vi "Process Inputs.vi"(10 "Command Inputs":T1, 11 "Sensor Inputs":T9) -> (3 "OutputsCluster":T16)   [LabVIEW 2012]
uses:
  Outputs_All.ctl
  Flywheel/Outputs_Flywheel.ctl
  tankdrive/Output_Wheel_Speeds.ctl
  Conveyor/Conveyor_outputs.ctl
  Conveyor/Conveyor module state.ctl
  Conveyor/Conveyor_outputsV2.ctl
  Conveyor/3-Ball-Conveyor_Module_State.ctl
  Conveyor/T_Roller module state.ctl
  Turret/Outputs_Turret.ctl
  Roller/Outputs_Roller.ctl
  Bridge Tipper/Outputs_Tipper.ctl
  Inputs_All.ctl
  Flywheel/Sensor_Inputs_FlyWheel.ctl
  tankdrive/Input_Sensors_Drive.ctl
  Conveyor/Sensor_Input_Conveyor.ctl
  Conveyor/Sensor_Input_ConveyorV2.ctl
  Turret/Inputs_Sensors_Turret.ctl
  Inputs_Camera.ctl
  Command_Inputs.ctl
  tankdrive/Input_Commands_Drive.ctl
  Conveyor/Input_Command_Conveyor.ctl
  Turret/Inputs_Commands_Turret.ctl
  Bridge Tipper/Inputs_Tipper.ctl
  Dashboard Controls.ctl
  Roller/Input_Commands_Roller.ctl
  Flywheel/Input_Commands_Flywheel.ctl
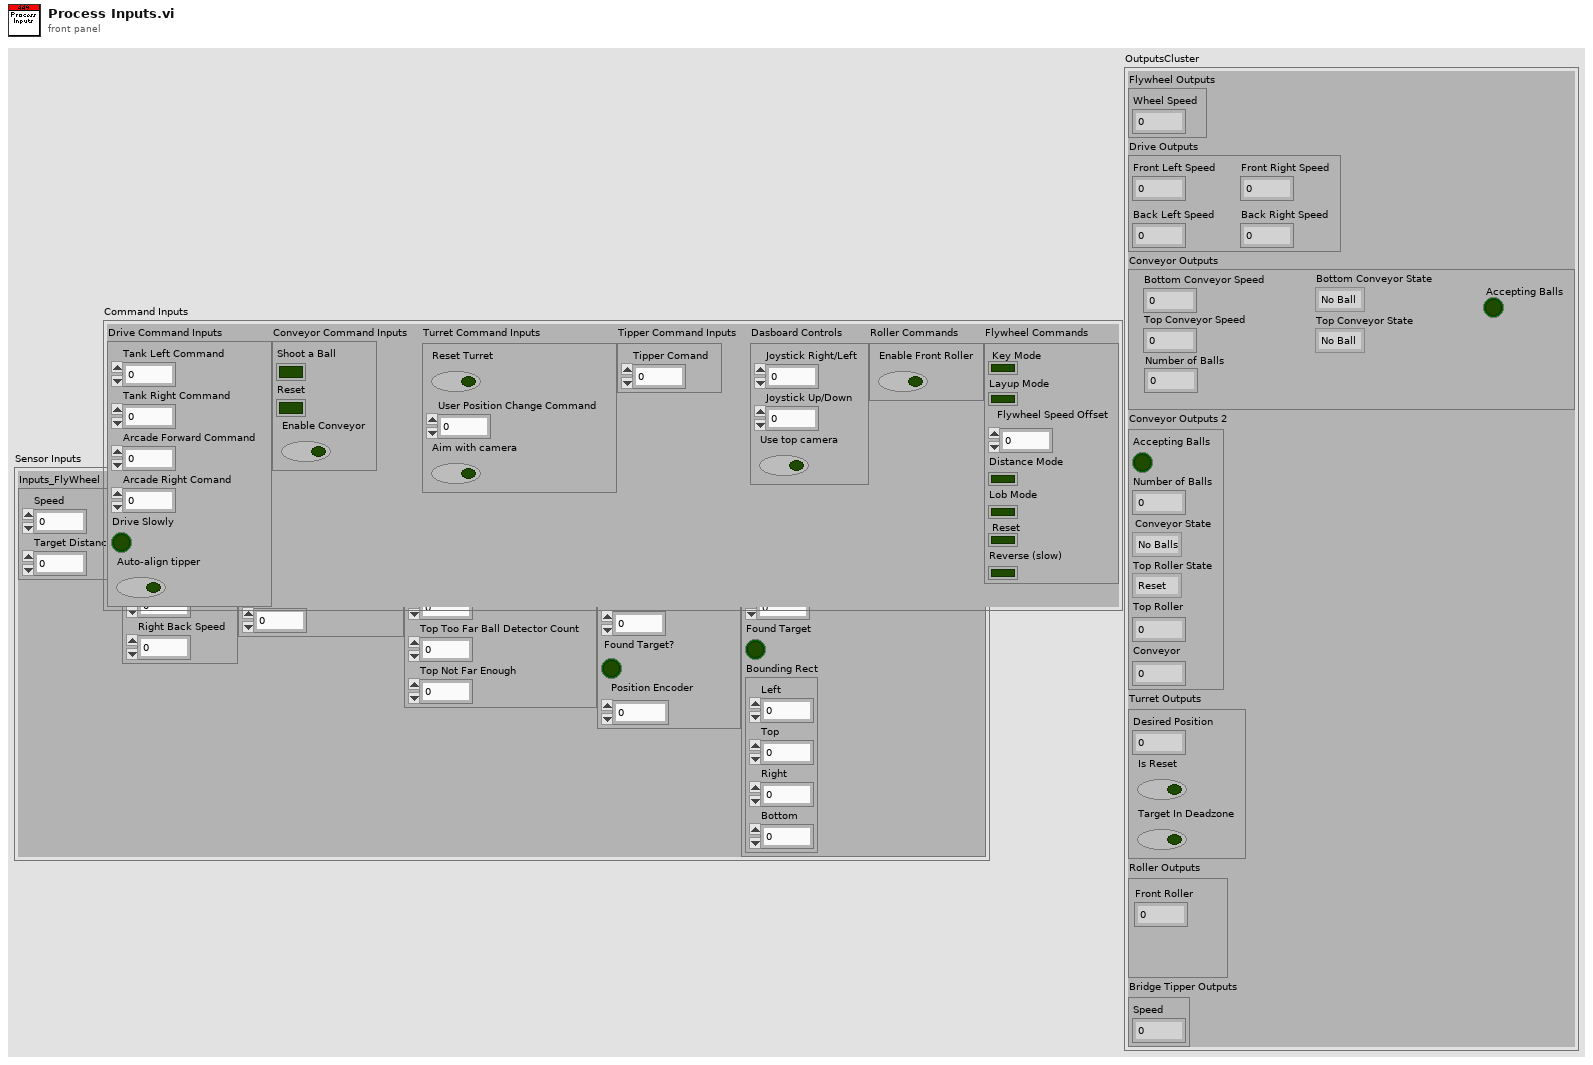
[diagram p1: front panel]
types:
  T1 = typedef "Command_Inputs.ctl" = cluster{"Drive Command Inputs":T2, "Conveyor Command Inputs":T3, "Turret Command Inputs":T4, "Tipper Command Inputs":T5, "Dasboard Controls":T6, "Roller Commands":T7, "Flywheel Commands":T8}
  T2 = typedef "Input_Commands_Drive.ctl" = cluster{"Tank Left Command":dbl, "Tank Right Command":dbl, "Arcade Forward Command":dbl, "Arcade Right Comand":dbl, "Drive Slowly":bool, "Auto-align tipper":bool}
  T3 = typedef "Input_Command_Conveyor.ctl" = cluster{"Shoot a Ball":bool, "Reset":bool, "Enable Conveyor":bool}
  T4 = typedef "Inputs_Commands_Turret.ctl" = cluster{"Reset Turret":bool, "User Position Change Command":dbl, "Aim with camera":bool}
  T5 = typedef "Inputs_Tipper.ctl" = cluster{"Tipper Comand":dbl}
  T6 = typedef "Dashboard Controls.ctl" = cluster{"Joystick Right/Left":dbl, "Joystick Up/Down":dbl, "Use top camera":bool}
  T7 = typedef "Input_Commands_Roller.ctl" = cluster{"Enable Front Roller":bool}
  T8 = typedef "Input_Commands_Flywheel.ctl" = cluster{"Key Mode":bool, "Layup Mode":bool, "Flywheel Speed Offset":dbl, "Distance Mode":bool, "Lob Mode":bool, "Reset":bool, "Reverse (slow)":bool}
  T9 = typedef "Inputs_All.ctl" = cluster{"Inputs_FlyWheel":T10, "Drive Inputs":T11, "Conveyor Inputs":T12, "ConveyorV2 Inputs":T13, "Turret Inputs":T14, "Camera Inputs":T15}
  T10 = typedef "Sensor_Inputs_FlyWheel.ctl" = cluster{"Speed":dbl, "Target Distance":dbl}
  T11 = typedef "Input_Sensors_Drive.ctl" = cluster{"Left Front Speed":dbl, "Right Front Speed":dbl, "Left Back Speed":dbl, "Right Back Speed":dbl}
  T12 = typedef "Sensor_Input_Conveyor.ctl" = cluster{"Top Ball Detector Count":i32, "Bottom Ball Detector Count":i32, "Shooter Ball Detector Count":i32}
  T13 = typedef "Sensor_Input_ConveyorV2.ctl" = cluster{"Grab Ball Detector Count":i32, "Bottom Ball Detector Count":i32, "Top In Place Ball Detector Count":i32, "Top Too Far Ball Detector Count":i32, "Top Not Far Enough":i32}
  T14 = typedef "Inputs_Sensors_Turret.ctl" = cluster{"At Minimum Angle":bool, "At Maximum Angle":bool, "Camera Position Offset":dbl, "Found Target?":bool, "Position Encoder":dbl}
  T15 = typedef "Inputs_Camera.ctl" = cluster{"Offset Angle from Perpendicular (degrees)":dbl, "Target Dist":dbl, "Elevation Angle":dbl, "Found Target":bool, "Bounding Rect":cluster{"Left":dbl, "Top":dbl, "Right":dbl, "Bottom":dbl}}
  T16 = typedef "Outputs_All.ctl" = cluster{"Flywheel Outputs":T17, "Drive Outputs":T18, "Conveyor Outputs":T19, "Conveyor Outputs 2":T21, "Turret Outputs":T24, "Roller Outputs":T25, "Bridge Tipper Outputs":T26}
  T17 = typedef "Outputs_Flywheel.ctl" = cluster{"Wheel Speed":dbl}
  T18 = typedef "Output_Wheel_Speeds.ctl" = cluster{"Front Left Speed":dbl, "Front Right Speed":dbl, "Back Left Speed":dbl, "Back Right Speed":dbl}
  T19 = typedef "Conveyor_outputs.ctl" = cluster{"Bottom Conveyor Speed":dbl, "Top Conveyor Speed":dbl, "Bottom Conveyor State":T20, "Top Conveyor State":T20, "Accepting Balls":bool, "Number of Balls":i32}
  T20 = typedef "Conveyor module state.ctl" = enum16{"No Ball", "Has Ball", "Ball Below Hold", "Ball Above Hold", "Outputting Ball", "Reset"}
  T21 = typedef "Conveyor_outputsV2.ctl" = cluster{"Accepting Balls":bool, "Number of Balls":i32, "Conveyor State":T22, "Top Roller State":T23, "Top Roller":dbl, "Conveyor":dbl}
  T22 = typedef "3-Ball-Conveyor_Module_State.ctl" = enum16{"No Balls", "Collecting Ball", "Holding 1", "Pushing Ball Out", "Holding 2", "Lowering Ball", "Reset", "Disabled"}
  T23 = typedef "T_Roller module state.ctl" = enum16{"Reset", "Disabled", "Waiting for Ball", "Holding", "Ball not far enough", "Ball too far", "Firing"}
  T24 = typedef "Outputs_Turret.ctl" = cluster{"Desired Position":dbl, "Is Reset":bool, "Target In Deadzone":bool}
  T25 = typedef "Outputs_Roller.ctl" = cluster{"Front Roller":dbl}
  T26 = typedef "Outputs_Tipper.ctl" = cluster{"Speed":dbl}
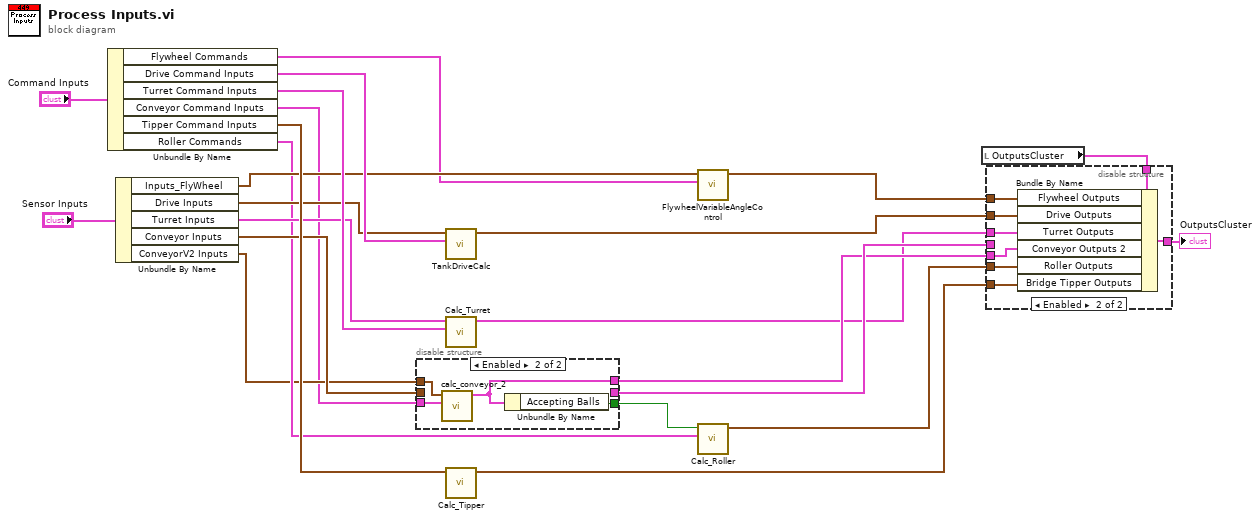
[diagram p0: block diagram]
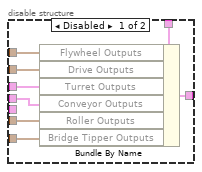
[diagram p2: hidden frame]
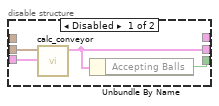
[diagram p3: hidden frame]
diagram:
  n1 = Unbundle By Name("Command Inputs") -> ("Flywheel Commands"=w7:T8, "Drive Command Inputs"=w17:T2, "Turret Command Inputs"=w19:T4, "Conveyor Command Inputs"=w2:T3, "Tipper Command Inputs"=w22:T5, "Roller Commands"=w6:T7)
  n2 = Unbundle By Name("Sensor Inputs") -> ("Inputs_FlyWheel"=w14:T10, "Drive Inputs"=w15:T11, "Turret Inputs"=w18:T14, "Conveyor Inputs"=w20:T12, "ConveyorV2 Inputs"=w5:T13)
  n3 = disable-structure shown="Enabled" {
    disable-tunnel: [w25 _] -> w23
    disable-tunnel: w2 -> [w27 w31]
    disable-tunnel: w20 -> [w26 _]
    disable-tunnel: w5 -> [_ w30]
    disable-tunnel: [_ w29] -> w3
    disable-tunnel: [w24 w28] -> w4
    frame Disabled {
      n4 = call "calc_conveyor.vi"("Conveyor Command Inputs"=w27, "Conveyor Sensor Inputs"=w26) -> ("Conveyor Outputs"=w25:T19)  [unwired: 9 in]
      n5 = Unbundle By Name(w25) -> ("Accepting Balls"=w24:bool)
    }
    frame Enabled {
      n6 = call "calc_conveyor_2.vi"("Conveyor Command Inputs"=w31, "ConveyorV2 Inputs"=w30) -> ("Conveyor Outputs"=w29:T21)  [unwired: 9 in]
      n7 = Unbundle By Name(w29) -> ("Accepting Balls"=w28:bool)
    }
  }
  n8 = call "TankDriveCalc.vi"("Drive Command Inputs"=w17, "Drive Sensor Inputs"=w15) -> ("Drive Outputs"=w10:T18)  [unwired: 9 in]
  n9 = call "Calc_Turret.vi"("Turret Command Inputs"=w19, "Turret Sensor Inputs"=w18) -> ("Turret Outputs"=w1:T24)  [unwired: 9 in]
  n10 = call "Calc_Tipper.vi"("Tipper Command Inputs"=w22) -> ("Bridge Tipper Outputs"=w13:T26)  [unwired: 10 in]
  n11 = call "FlywheelVariableAngleControl.vi"("Flywheel Commands"=w7, "Inputs_FlyWheel"=w14) -> ("Outputs_Flywheel"=w9:T17)  [unwired: 9 in]
  n12 = call "Calc_Roller.vi"("Roller Commands"=w6, "Accepting Balls?"=w4) -> ("Roller Outputs"=w12:T25)  [unwired: 9 in]
  n13 = local read "OutputsCluster"() -> (w8:T16)
  n14 = disable-structure shown="Enabled" {
    disable-tunnel: w1 -> [w39 w43]
    disable-tunnel: w23 -> [w38 _]
    disable-tunnel: w13 -> [w37 w41]
    disable-tunnel: w12 -> [w36 w42]
    disable-tunnel: [w35 w47] -> w11
    disable-tunnel: w10 -> [w34 w44]
    disable-tunnel: w9 -> [w33 w45]
    disable-tunnel: w8 -> [w32 w46]
    disable-tunnel: w3 -> [_ w40]
    frame Disabled {
      n15 = Bundle By Name(cluster=w32, "Flywheel Outputs"=w33, "Drive Outputs"=w34, "Turret Outputs"=w39, "Conveyor Outputs"=w38, "Roller Outputs"=w36, "Bridge Tipper Outputs"=w37) -> (w35:T16)
    }
    frame Enabled {
      n16 = Bundle By Name(cluster=w46, "Flywheel Outputs"=w45, "Drive Outputs"=w44, "Turret Outputs"=w43, "Conveyor Outputs 2"=w40, "Roller Outputs"=w42, "Bridge Tipper Outputs"=w41) -> (w47:T16)
    }
  }
  "OutputsCluster" <- w11
